vi "Dashboard Main.vi"() -> ()   [LabVIEW 2023]
uses:
  <vilib>/event_ctls.llb/eventvkey.ctl
  <vilib>/Rock Robotics/Network Tables/NT Read Numeric Array.vi
  <vilib>/Rock Robotics/WPI/Dashboard/WPI_DashboardLogging Global.vi
panel:
  in  "Camera Settings Right":T1={"Frame Rate"=30, "Compression"=30, "Size"=1, "DB Camera Config"=FALSE} {"Frame Rate" scale=1.0..30.0; "Compression" scale=100.0..-1.0; "Size" items=["640x480", "320x240", "160x120"]}
  in  "Camera Name Right":string(combo)="No Camera Selection"
  out "Camera Perf":string
  in  "Camera Settings":T1={"Frame Rate"=30, "Compression"=30, "Size"=1, "DB Camera Config"=FALSE} {"Frame Rate" scale=1.0..30.0; "Compression" scale=100.0..-1.0; "Size" items=["640x480", "320x240", "160x120"]}
  in  "TCP":refnum<k5>
  in  "Rec Mode":enum32{"Stop", "Record", "Playback"}(radio)
  out "Robot IP":string
  out "Image Message":string="Timeout in Camera Communications"
  in  "Dashboard Tab":T2(tab)
  in  "Select Auto":string(combo)="Select Autonomous ..."
  out "NT Connection":bool
  out "MotorChart R":cluster{"Numeric":dbl, "Numeric":dbl}(graph)
  out "MotorChart L":cluster{"Numeric":dbl, "Numeric":dbl}(graph)
  out "MotorSliders R":cluster{"MotorSlide1":dbl, "MotorSlide2":dbl} {"MotorSlide2" scale=-1.0..1.0 scale format="%#_2e"; "MotorSlide1" scale=-1.0..1.0 scale format="%#_2e"}
  out "MotorSliders L":cluster{"MotorSlide1":dbl, "MotorSlide2":dbl} {"MotorSlide2" scale=-1.0..1.0 scale format="%#_2e"; "MotorSlide1" scale=-1.0..1.0 scale format="%#_2e"}
  out "Encoder":dbl(knob) scale=0.0..360.0
  out "JS1 Z":dbl(slide) scale=-1.0..1.0 scale format="%#_2e"
  out "JS1 Graph":cluster{"X":dbl, "Y":dbl}[](graph)
  out "JS1 Buttons":T3
  out "JS2 Z":dbl(slide) scale=-1.0..1.0 scale format="%#_2e"
  out "JS2 Graph":cluster{"X":dbl, "Y":dbl}[](graph)
  out "JS2 Buttons":T3
  out "Mode":T4(ring)=enum."Auto Disabled"
  out "Right Camera Perf":cluster{"Bandwidth (Mbps)":dbl, "FPS":dbl}
  out "Camera Image Right":T5(plugin-control)
  in  "DB/String 9":string
  in  "DB/String 8":string
  in  "DB/String 7":string
  in  "DB/String 6":string
  in  "DB/String 5":string
  in  "DB/String 4":string
  in  "DB/String 3":string
  in  "DB/String 2":string
  in  "DB/String 1":string
  in  "DB/String 0":string
  in  "DB/Slider 0":dbl(slide) scale=0.0..5.0
  in  "DB/Slider 1":dbl(slide) scale=0.0..5.0
  in  "DB/Slider 2":dbl(slide) scale=0.0..5.0
  in  "DB/Slider 3":dbl(slide) scale=0.0..5.0
  out "DB/LED 3":bool
  out "DB/LED 2":bool
  out "DB/LED 1":bool
  out "DB/LED 0":bool
  in  "DB/Button 3":bool
  in  "DB/Button 2":bool
  in  "DB/Button 1":bool
  in  "DB/Button 0":bool caption="New Name"
  out "valorMotorEncoder":dbl
  out "encoderPsAlga":dbl(knob) scale=0.0..360.0
  in  "Test Slider":dbl(slide) scale=0.0..100.0 scale format="%#_3g"
  in  "On/Off":bool caption="Solenoid"
  in  "Test Name":u16(ring) items=["Select the test to run..."]
  in  "Test Tree":string(tree)
  in  "Motor":cluster{"Value":dbl, "Enable":bool} {"Value" scale=-1.0..1.0 scale format="%#_3g"}
  out "Progress":T6 {"Test Progress" scale=0.0..100.0}
  in  "Rev/Fwd":cluster{"Forward":bool, "Reverse":bool}
  in  "Test Ring":u16(ring) items=["Monochrome", "Color"]
  in  "CheckList":i32(listbox)
  out "Tree":string(tree)
  out "Camera Image":T5(plugin-control)
  out "Background":bool
  in  "Camera Name":string(combo)="No Camera Selection"
  # "HW"
  # "HW"
  # "Joysticks"
  # "Motores"
  # "Front"
  # "Right"
  # "Left"
  # "Back"
  # "Encoder"
  # "Valor do encoder (dado em rotações)"
  # "Valor do motor"
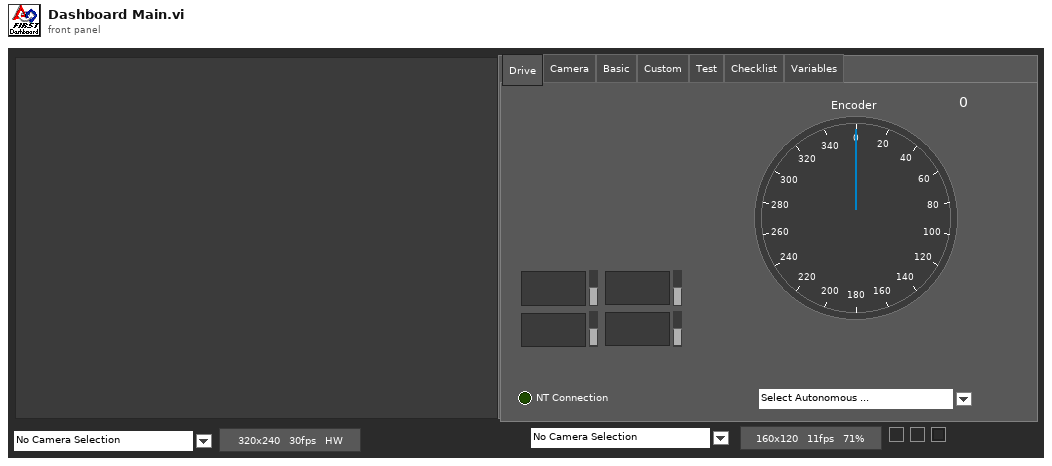
[diagram p1: front panel]
types:
  T1 = cluster{"Frame Rate":i32, "Compression":i32, "Size":u16, "DB Camera Config":bool}
  T2 = enum32{"Drive", "Camera", "Basic", "Custom", "Test", "Checklist", "Variables"}
  T3 = cluster{bool, bool, bool, bool, bool, bool, bool, bool, bool, bool, bool, bool}
  T4 = enum8{"Tele-Op Disabled", "Tele-Op Enabled", "Auto Disabled", "Auto Enabled", "Test Disabled", "Test Enabled", "Disconnected", "No Code", "E-Stop"}
  T5 = typedef "IMAQ Image.ctl" = refnum<image>
  T6 = cluster{"Test Progress":u8, "Test Progress Text":string}
  T7 = cluster{"Save Path":path, "Interval (s)":dbl, "Keep":i32}
  T8 = enum32{"Drive", "Camera", "Basic", "Custom", "Test", "Commands", "Checklist", "Variables"}
  T9 = typedef "Image Type" = u32
  T10 = cluster{"Error Strings":string, "Disable Counts":cluster{u16, u16}, "Rail Faults":cluster{u16, u16, u16}, "Robot IP":string, "DB Mode":u8, "Event Info":cluster{"Name":string, "Type":u8, "Number":u16, "Replay":u8}}
  T11 = cluster{"Storage":cluster{"Disk Free":u64, "RAM Block":u32, "RAM free":u32}, "CPU Utilization":cluster{"CPU % ISR":sgl, "CPU % Time Crit":sgl, "CPU % Timed Str":sgl, "CPU % High":sgl, "CPU % Above":sgl, "CPU % Normal":sgl, "CPU % Low":sgl}, "CAN":cluster{"% Bus Utilization":sgl, "Bus Off Cnt":u32, "TX_FIFO Full Cnt":u32, "Receive Error Cnt":u8, "Transmit Error Cnt":u8}, "HID":cluster{"HID Outputs":u32, "Rumble Low":u16, "Rumble High":u16}[]}
  T12 = cluster{"Status bits":cluster{"Test Mode":bool, "Autonomous":bool, "Enabled":bool, "Code Start":bool, "Brownout":bool, "Reserved 2":bool, "Reserved 3":bool, "E-Stop":bool}, "Code Trace":cluster{"Disabled":bool, "TeleOp":bool, "Auto":bool, "Test":bool}, "Controller Type":enum16{"unknown", "cRIO", "roboRio"}, "Code?":enum16{"unknown", "noCode", "code"}, "Battery V":dbl}
  T13 = cluster{"Control Bits":cluster{"TestMode":bool, "Autonomous":bool, "Enabled":bool, "FMS Present":bool, bool, bool, bool, "E-Stop":bool}, "Team Station ":u8, "Countdown":sgl, "Joystick Values":cluster{"Axes":dbl[], "Buttons":bool[], "POVs":i16[]}[]}
  T14 = cluster{"Axes":dbl[], "Buttons":bool[], "POVs":i16[]}[]
  T15 = cluster{"Axes":dbl[], "Buttons":bool[], "POVs":i16[]}
  T16 = cluster{"Buttons[0]":bool, "Buttons[1]":bool, "Buttons[2]":bool, "Buttons[3]":bool, "Buttons[4]":bool, "Buttons[5]":bool, "Buttons[6]":bool, "Buttons[7]":bool, "Buttons[8]":bool, "Buttons[9]":bool, "Buttons[10]":bool, "Buttons[11]":bool}
  T17 = cluster{"Camera Image":refnum<vi>, "Dashboard Tab":refnum<vi>, "Background":refnum<vi>, "Rec Mode":refnum<vi>, "Test Slider":refnum<vi>, "On/Off ":refnum<vi>, "Test Ring":refnum<vi>, "Rev/Fwd":refnum<vi>, "Test Name":refnum<vi>, "Motor":refnum<vi>, "Progress":refnum<vi>, "CheckList":refnum<vi>, "Tree":refnum<vi>, "Test Tree":refnum<vi>, "Camera Settings":refnum<vi>, "Camera Name":refnum<vi>, "Camera Perf":refnum<vi>, "Camera Settings Right":refnum<vi>, "Camera Name Right":refnum<vi>, "Camera Image Right":refnum<vi>}
  T18 = cluster{"Global Rectangle":i32[], "Contours":cluster{"Contour Type":u32, "ROI Type":u32, "Points":i32[]}[]}
  T19 = cluster{"Camera Name":string, string, "Saved DB Images Info":cluster{"Save Path":path, "Interval (s)":dbl, "Keep":i32}}
  T20 = cluster{"Camera Name Right":string, string, "Saved DB Images Info":cluster{"Save Path":path, "Interval (s)":dbl, "Keep":i32}}
  T21 = cluster{"Operation":enum16{"Update", "Clear"}, "Color Box":u32}[]
  T22 = typedef "eventvkey.ctl" = enum16{"ASCII", "Enter", "Return", "Shift", "Ctrl", "Alt", "Cmd", "Opt", "Caps", "NumLock", "Clear", "Break", "Up", "Down", "Left", "Right", "Insert", "Delete", "Home", "End", "PageUp", "PageDown", "Escape", "Help", "Pause", "ScrollLock", "F1", "F2", "F3", "F4", "F5", "F6", "F7", "F8", "F9", "F10", "F11", "F12", "F13", "F14", "F15", "F16", "F17", "F18", "F19", "F20", "F21", "F22", "F23", "F24", "Play", "VolumeUp", "VolumeDown", "Mute", "Two Byte Char"}
  T23 = cluster{"Image Size":bool, "Image Type":bool, "Pixel Value":bool, "ROI Information":bool, "Zoom Factor":bool}
  T24 = cluster{"Operation":enum16{"Update", "Clear"}, "Color Box":u32}
  T25 = cluster{"Shift":bool, "Ctrl":bool, "Alt":bool, "Cmd":bool, "Opt":bool}
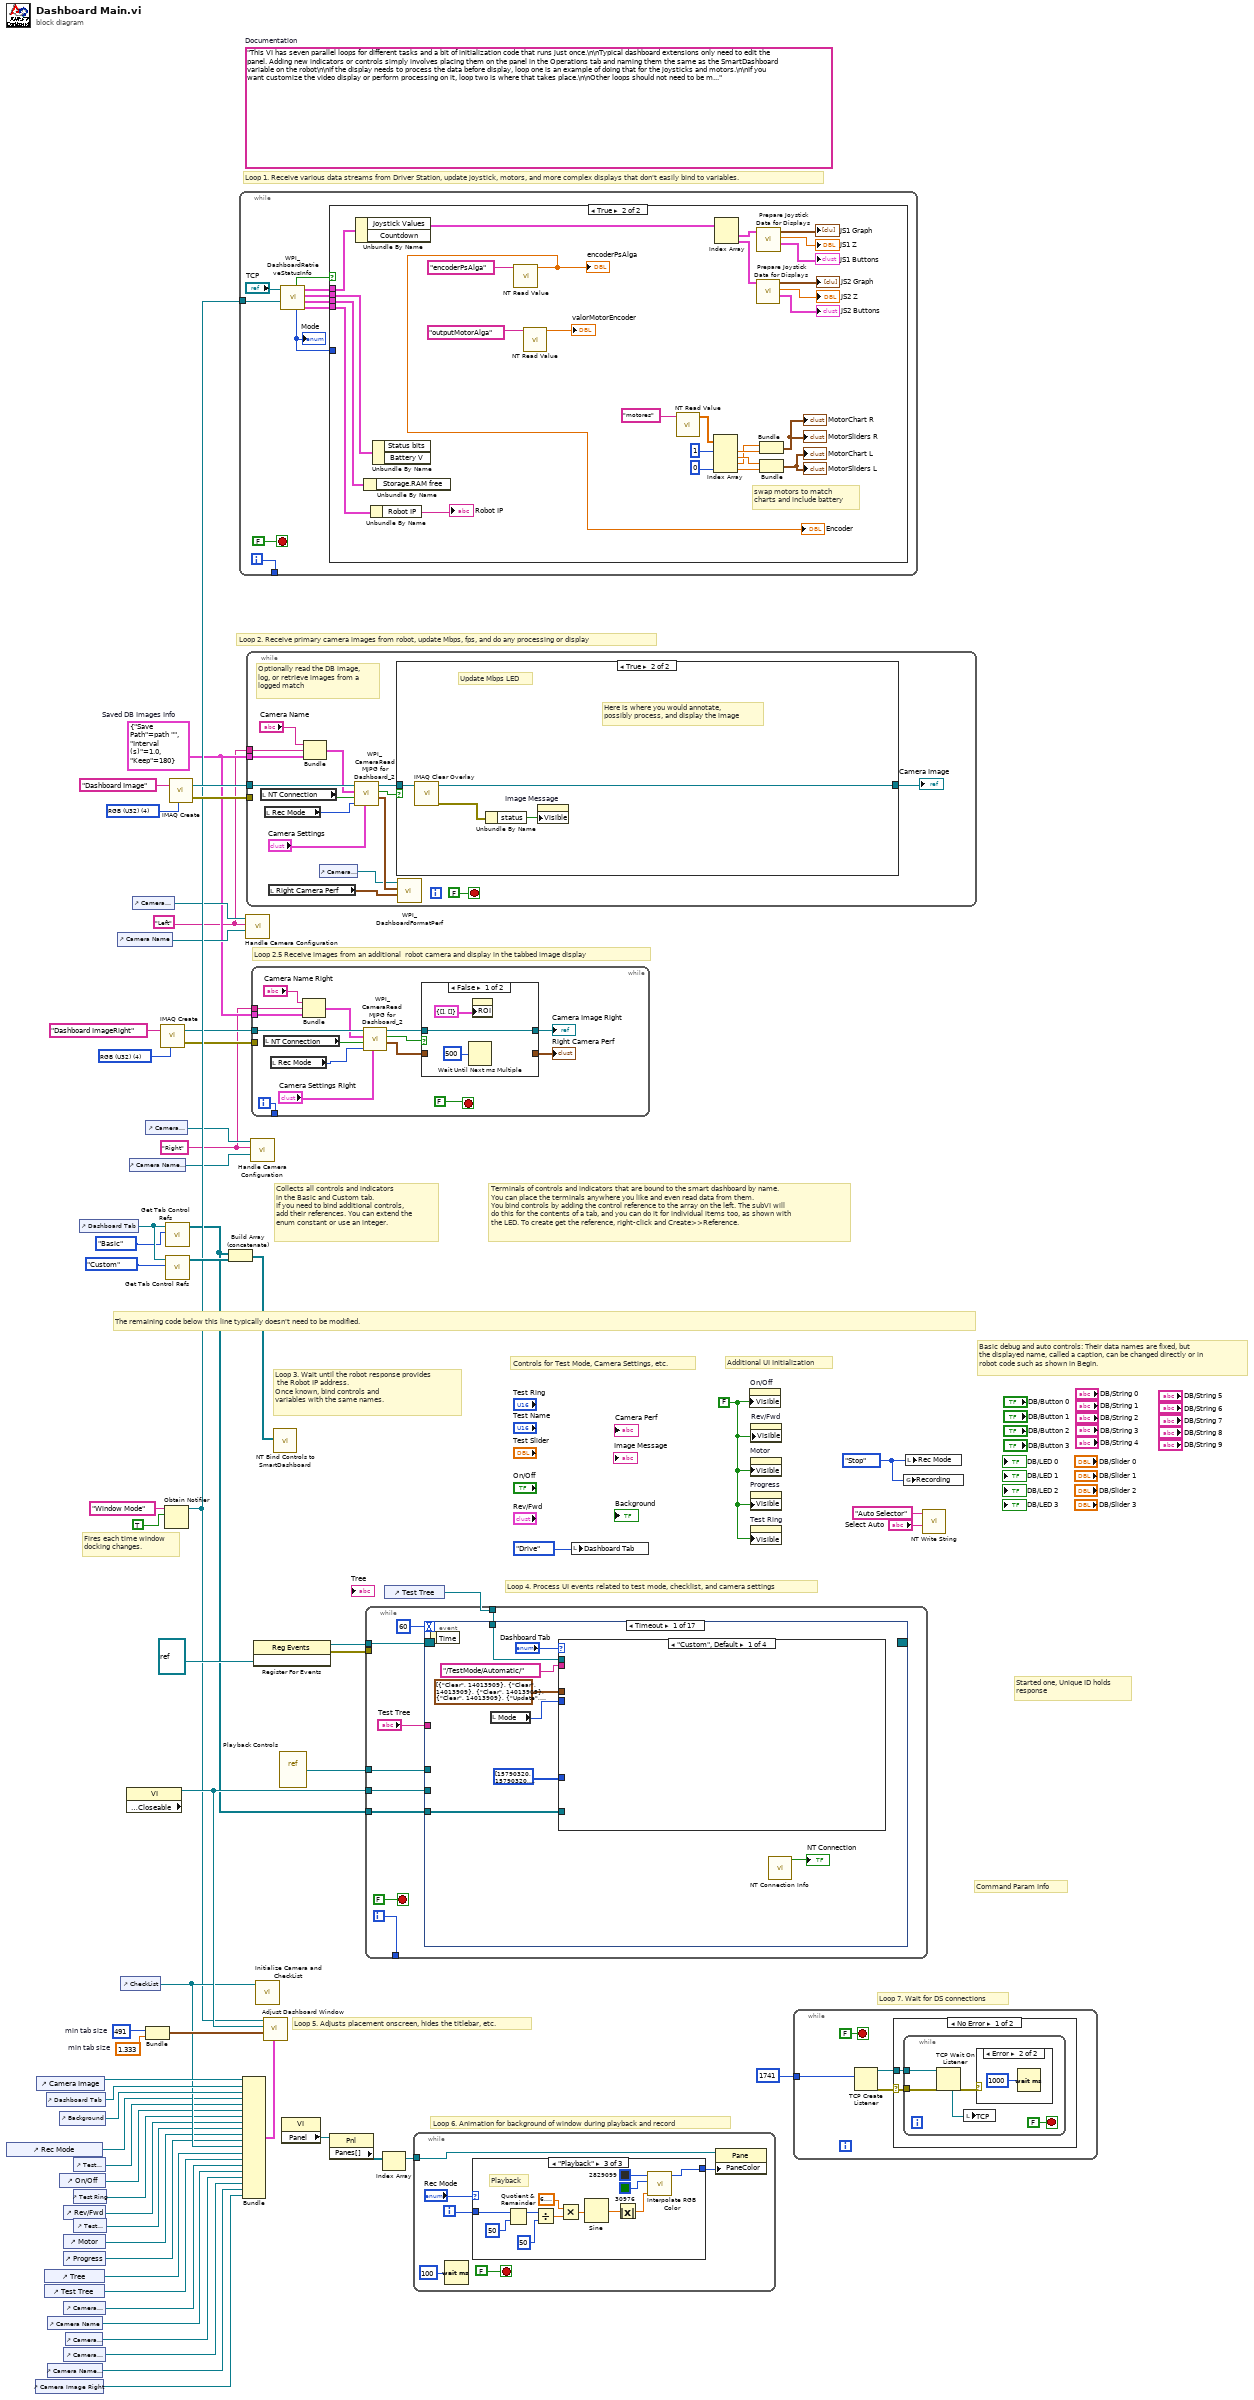
[diagram p0: block diagram]
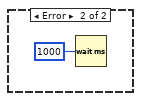
[diagram p4: hidden frame]
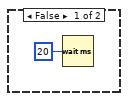
[diagram p5: hidden frame]
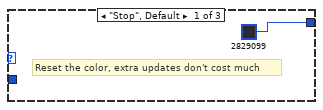
[diagram p6: hidden frame]
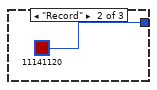
[diagram p7: hidden frame]
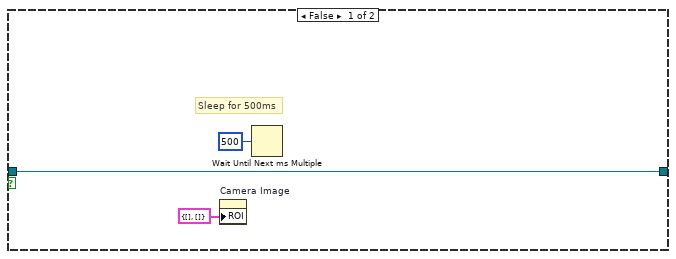
[diagram p8: hidden frame]
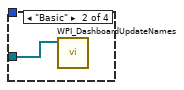
[diagram p9: hidden frame]
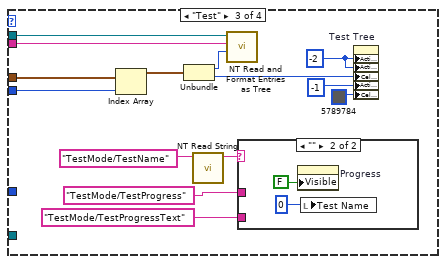
[diagram p10: hidden frame]
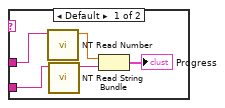
[diagram p11: hidden frame]
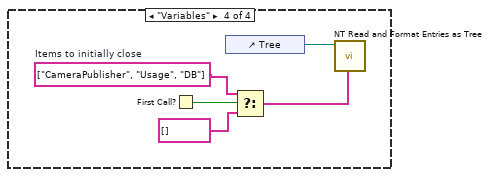
[diagram p12: hidden frame]
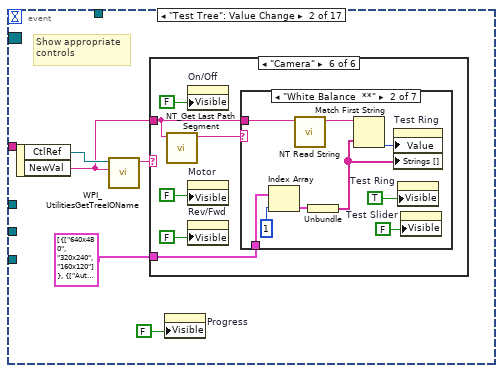
[diagram p13: hidden frame]
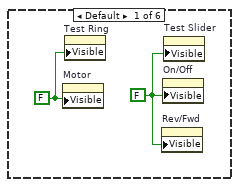
[diagram p14: hidden frame]
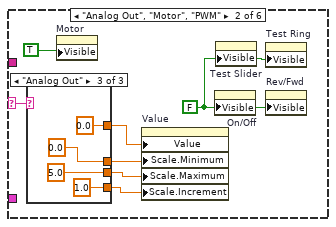
[diagram p15: hidden frame]
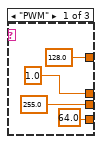
[diagram p16: hidden frame]
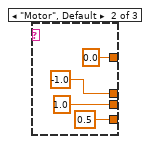
[diagram p17: hidden frame]
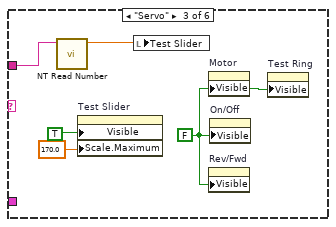
[diagram p18: hidden frame]
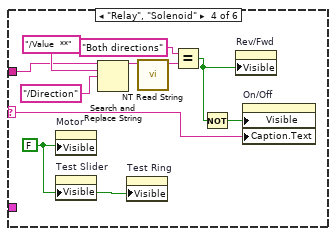
[diagram p19: hidden frame]
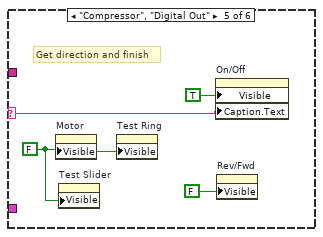
[diagram p20: hidden frame]
diagram:
  w3 = T7 {"Save Path"=path "", "Interval (s)"=1.0, "Keep"=180}  # Saved DB Images Info
  w2 = "Right"
  w1 = "Left"
  w13 = T9 4 items=["Grayscale (U8)", "Grayscale (I16)", "Grayscale (SGL)", "Complex (CSG)", "RGB (U32)", "HSL (U32)", "RGB (U64)"] ("Image Type")
  w42 = 491  # min tab size
  w41 = 1.333  # min tab size
  w49 = enum32{"Stop", "Record", "Playback"}."Stop" ("Rec Mode")
  w26 = FALSE ("Visible")
  (unwired) "This VI has seven parallel loops for different tasks and a bit of initialization code that runs just once.\n\nTypical dashboard extensions only need to edit the panel. Adding new indicators or controls simply involves placing them on the panel in the Operations tab and naming them the same as the SmartDashboard variable on the robot\n\nIf the display needs to process the data before display, loop one is an example of doing that for the joysticks and motors.\n\nIf you want customize the video display or perform processing on it, loop two is where that takes place.\n\nOther loops should not need to be modified. They are pretty standard, and document the task they perform."  # Documentation
  w63 = T9 4 items=["Grayscale (U8)", "Grayscale (I16)", "Grayscale (SGL)", "Complex (CSG)", "RGB (U32)", "HSL (U32)", "RGB (U64)"] ("Image Type")
  # "Loop 2.5 Receive images from an additional  robot camera and display in the tabbed image display"
  # "Command Param Info"
  # "Started one, Unique ID holds\nresponse"
  # "Loop 7. Wait for DS connections"
  # "Basic debug and auto controls: Their data names are fixed, but\nthe displayed name, called a caption, can be changed directly or in\nrobot code such as shown in Begin."
  # "Controls for Test Mode, Camera Settings, etc."
  # "Additional UI Initialization"
  # "Loop 6. Animation for background of window during playback and record"
  # "Fires each time window\ndocking changes."
  # "Collects all controls and indicators\nin the Basic and Custom tab.\nIf you need to bind additional controls,\nadd their references. You can extend the\nenum constant or use an integer."
  # "The remaining code below this line typically doesn't need to be modified."
  # "Loop 4. Process UI events related to test mode, checklist, and camera settings"
  # "Terminals of controls and indicators that are bound to the smart dashboard by name.\nYou can place the terminals anywhere you like and even read data from them.\nYou bind controls by adding the control reference to the array on the left. The subVI will\ndo this for the contents of a tab, and you can do it for individual items too, as shown with\nthe LED. To create get the reference, right-click and Create>>Reference."
  # "Loop 3. Wait until the robot response provides\n the Robot IP address.\nOnce known, bind controls and\nvariables with the same names."
  # "Loop 5. Adjusts placement onscreen, hides the titlebar, etc."
  # "Loop 1. Receive various data streams from Driver Station, update joystick, motors, and more complex displays that don't easily bind to variables."
  # "Loop 2. Receive primary camera images from robot, update Mbps, fps, and do any processing or display"
  n1 = control-ref of="Rec Mode"() -> (w32:refnum<vi>)
  n2 = control-ref of="Camera Image Right"() -> (w6:refnum<vi>)
  n3 = control-ref of="Camera Image"() -> (w44:refnum<vi>)
  n4 = control-ref of="Tree"() -> (w36:refnum<vi>)
  n5 = control-ref of="Test Tree"() -> (w35:refnum<vi>)
  n6 = control-ref of="Dashboard Tab"() -> (w43:refnum<vi>)
  n7 = control-ref of="Camera Name"() -> (w19:refnum<vi>)
  n8 = control-ref of="Camera Name Right"() -> (w7:refnum<vi>)
  n9 = control-ref of="Background"() -> (w39:refnum<vi>)
  n10 = control-ref of="On/Off"() -> (w30:refnum<vi>)
  n11 = control-ref of="Progress"() -> (w27:refnum<vi>)
  n12 = control-ref of="Camera Settings"() -> (w20:refnum<vi>)
  n13 = control-ref of="Camera Settings Right"() -> (w8:refnum<vi>)
  n14 = control-ref of="Rev/Fwd"() -> (w28:refnum<vi>)
  n15 = control-ref of="Motor"() -> (w33:refnum<vi>)
  n16 = control-ref of="Camera Perf"() -> (w18:refnum<vi>)
  n17 = control-ref of="Test Slider"() -> (w31:refnum<vi>)
  n18 = control-ref of="Test Ring"() -> (w29:refnum<vi>)
  n19 = control-ref of="Test Name"() -> (w34:refnum<vi>)
  n20 = control-ref of="Dashboard Tab"() -> (w47:refnum<vi>)
  n21 = control-ref of="Camera Name"() -> (w21:refnum<vi>)
  n22 = control-ref of="CheckList"() -> (w37:refnum<vi>)
  n23 = property class="VI" props=["Front Panel.Closeable"]() -> (reference out=w48:refnum<vi>)  [unwired: 2 in, 2 out]
  n24 = control-ref of="Camera Name Right"() -> (w9:refnum<vi>)
  n25 = control-ref of="Camera Settings"() -> (w22:refnum<vi>)
  n26 = control-ref of="Camera Settings Right"() -> (w10:refnum<vi>)
  n27 = Bundle("min tab size"=w42, "min tab size"=w41) -> (w40:cluster{"min tab size":i32, "min tab size":dbl})  [unwired: 1 in]
  n28 = call "IMAQ Create"("Image Name"="Dashboard ImageRight", "Image Type"=w13) -> ("New Image"=w12:T5, "error out"=w11:errorcluster)  [unwired: 2 in, 1 out]
  n29 = Obtain Notifier(name (unnamed)="Window Mode", notification data type=TRUE) -> (notifier out=w25:refnum<notifier>)  [unwired: 2 in, 2 out]
  n30 = call <vilib>:"Get Tab Control Refs.vi"("Page Index"=T8."Basic" ("Dashboard Tab"), "TabControl in"=w47) -> ("ControlsOnPage"=w17:refnum<vi>[])  [unwired: 9 in]
  n31 = call <vilib>:"Get Tab Control Refs.vi"("Page Index"=T8."Custom" ("Dashboard Tab"), "TabControl in"=w47) -> ("ControlsOnPage"=w46:refnum<vi>[])  [unwired: 9 in]
  n32 = call "IMAQ Create"("Image Name"="Dashboard Image", "Image Type"=w63) -> ("New Image"=w61:T5, "error out"=w60:errorcluster)  [unwired: 2 in, 1 out]
  n33 = Build Array (concatenate)(w17, w46) -> (w45:refnum<vi>[])
  n34 = while {
    tunnel: [w72] -> _
    tunnel: w25 -> [w64]
    i -> [w72]
    stop <- FALSE stop-if-true
    n35 = call <vilib>:"WPI_DashboardRetrieveStatusInfo.vi"("Window Mode Notifier"=w64, "TCP Cnx"="TCP") -> ("Power and Errors"=w67:T10, "Robot Metrics"=w70:T11, "Status Info"=w71:T12, "Control Info"=w68:T13, "Robot Mode"=w66:T4, "Process?"=w69:bool)  [unwired: 4 in]
    "Mode" <- w66
    n36 = case shown="True" w69 {
      tunnel: w71 -> [_ w102]
      tunnel: w70 -> [_ w101]
      tunnel: w68 -> [_ w100]
      tunnel: w67 -> [_ w99]
      tunnel: w66 -> [_ _]
      frame False {
        n37 = Wait (ms)(milliseconds to wait=u32 20) -> ()  [unwired: 1 out]
      }
      frame True {
        # "swap motors to match\ncharts and include battery"
        n38 = Unbundle By Name(w100) -> ("Joystick Values"=w90:T14)  [unwired: 1 out]
        n39 = Unbundle By Name(w101) -> ()  [unwired: 1 out]
        n40 = Unbundle By Name(w99) -> ("Robot IP"=→"Robot IP":string)
        n41 = Unbundle By Name(w102) -> ()  [unwired: 2 out]
        n42 = call-poly <vilib>:"NT Read Value.vi"("name"="encoderPsAlga") -> ("value"=→"Encoder" →"encoderPsAlga":dbl)  [unwired: 8 in, 2 out]
        n43 = call-poly <vilib>:"NT Read Value.vi"("name"="outputMotorAlga") -> ("value"=→"valorMotorEncoder":dbl)  [unwired: 8 in, 2 out]
        n44 = call-poly <vilib>:"NT Read Value.vi"("name"="motores" ("Name")) -> ("value"=w80:dbl[])  [unwired: 8 in, 2 out]
        n45 = Index Array(array=w80, index #1=1, index #4=0) -> (element #1=w94:dbl, element #2=w95:dbl, element #3=w93:dbl, element #4=w98:dbl)  [unwired: 2 in]
        n46 = Index Array(array=w90) -> (element #1=w89:T15, element #2=w85:T15)  [unwired: 2 in]
        n47 = call "Prepare Joystick Data for Displays.vi"("Joystick Values"=w85) -> ("Buttons"=→"JS2 Buttons":T16, "Z Axis"=→"JS2 Z":dbl, "Cartesian Data"=→"JS2 Graph":cluster{"X axis":dbl, "X axis":dbl}[])  [unwired: 8 in]
        n48 = call "Prepare Joystick Data for Displays.vi"("Joystick Values"=w89) -> ("Buttons"=→"JS1 Buttons":T16, "Z Axis"=→"JS1 Z":dbl, "Cartesian Data"=→"JS1 Graph":cluster{"X axis":dbl, "X axis":dbl}[])  [unwired: 8 in]
        n49 = Bundle("Numeric"=w93, "Numeric"=w94) -> (→"MotorChart R" →"MotorSliders R":cluster{"Numeric":dbl, "Numeric":dbl})  [unwired: 1 in]
        n50 = Bundle("Numeric"=w95, "Numeric"=w98) -> (→"MotorChart L" →"MotorSliders L":cluster{"Numeric":dbl, "Numeric":dbl})  [unwired: 1 in]
      }
    }
  }
  n51 = Bundle("Camera Image"=w44, "Dashboard Tab"=w43, "Background"=w39, "Rec Mode"=w32, "Test Slider"=w31, "On/Off"=w30, "Test Ring"=w29, "Rev/Fwd"=w28, "Test Name"=w34, "Motor"=w33, "Progress"=w27, "CheckList"=w37, "Tree"=w36, "Test Tree"=w35, "Camera Settings"=w20, "Camera Name"=w19, "Camera Perf"=w18, "Camera Settings Right"=w8, "Camera Name Right"=w7, "Camera Image Right"=w6) -> (w38:T17)  [unwired: 1 in]
  n52 = call "Handle Camera Configuration.vi"("CameraNameRef"=w21, "Display Name"=w1, "ClusterRef"=w22) -> ()  [unwired: 9 in]
  n53 = while {
    tunnel: w61 -> [w116]
    tunnel: w60 -> [_]
    tunnel: w3 -> [w109]
    tunnel: w1 -> [w106]
    stop <- FALSE stop-if-true
    # "Optionally read the DB image,\nlog, or retrieve images from a\nlogged match"
    n54 = local read "NT Connection"() -> (w110:bool)
    n55 = local read "Rec Mode"() -> (w113:enum32{"Stop", "Record", "Playback"})
    n56 = local read "Right Camera Perf"() -> (w104:cluster{"Bandwidth (Mbps)":dbl, "FPS":dbl})
    n57 = Bundle("Camera Name"="Camera Name", w106, "Saved DB Images Info"=w109) -> (w108:T19)  [unwired: 1 in]
    n58 = control-ref of="Camera Perf"() -> (w103:refnum<vi>)
    n59 = call <vilib>:"WPI_CameraRead MJPG for Dashboard_2.vi"("Camera Settings"="Camera Settings", "Rec Mode"=w113, "NT Connection"=w110, "Capture Info"=w108, "Image in"=w116) -> ("perf info"=w105:cluster{"Bandwidth (Mbps)":dbl, "fps":dbl}, "Active"=w114:bool, "Image\\ out"=w115:T5)  [unwired: 4 in]
    n60 = case shown="True" w114 {
      tunnel: w115 -> [w119 w122]
      tunnel: [w119 w121] -> w111
      frame False {
        # "Sleep for 500ms"
        n61 = property on="Camera Image" class="ImageControl"("ROI"=T18 {"Global Rectangle"=[], "Contours"=[]}) -> ()  [unwired: 2 in, 2 out]
        n62 = Wait Until Next ms Multiple(millisecond multiple=u32 500) -> ()  [unwired: 1 out]
      }
      frame True {
        # "Here is where you would annotate,\npossibly process, and display the image"
        # "Update Mbps LED"
        n63 = call "IMAQ Clear Overlay"("Image"=w122) -> ("error out"=w123:errorcluster, "Image Out"=w121:T5)  [unwired: 2 in, 7 out]
        n64 = Unbundle By Name(w123) -> ("status"=w124:bool)
        n65 = property on="Image Message" class="Str"("Visible"=w124) -> ()  [unwired: 2 in, 2 out]
      }
    }
    "Camera Image" <- w111
    n66 = call <vilib>:"WPI_DashboardFormatPerf.vi"("Right Camera Perf"=w104, "Performance"=w105, "String in"=w103) -> ()  [unwired: 9 in]
  }
  n67 = call "Handle Camera Configuration.vi"("CameraNameRef"=w9, "Display Name"=w2, "ClusterRef"=w10) -> ()  [unwired: 9 in]
  n68 = while {
    tunnel: w12 -> [w139]
    tunnel: w11 -> [_]
    tunnel: [w134] -> _
    tunnel: w3 -> [w130]
    tunnel: w2 -> [w127]
    i -> [w134]
    stop <- FALSE stop-if-true
    n69 = local read "NT Connection"() -> (w131:bool)
    n70 = local read "Rec Mode"() -> (w138:enum32{"Stop", "Record", "Playback"})
    n71 = Bundle("Camera Name Right"="Camera Name Right", w127, "Saved DB Images Info"=w130) -> (w129:T20)  [unwired: 1 in]
    n72 = call <vilib>:"WPI_CameraRead MJPG for Dashboard_2.vi"("Camera Settings"="Camera Settings Right", "Rec Mode"=w138, "NT Connection"=w131, "Capture Info"=w129, "Image in"=w139) -> ("perf info"=w125:cluster{"Bandwidth (Mbps)":dbl, "fps":dbl}, "Active"=w133:bool, "Image\\ out"=w136:T5)  [unwired: 4 in]
    n73 = case shown="False" w133 {
      tunnel: w136 -> [w141 w144]
      tunnel: [w141 w144] -> w132
      tunnel: [_ w143] -> w126
      tunnel: w125 -> [_ w143]
      frame False {
        n74 = Wait Until Next ms Multiple(millisecond multiple=u32 500) -> ()  [unwired: 1 out]
        n75 = property on="Camera Image Right" class="ImageControl"("ROI"=T18 {"Global Rectangle"=[], "Contours"=[]}) -> ()  [unwired: 2 in, 2 out]
      }
      frame True {
      }
    }
    "Camera Image Right" <- w132
    "Right Camera Perf" <- w126
  }
  n76 = register-events(refnum<vi> refnum) -> (reference out=w52:refnum<event-registration>, error out=w51:errorcluster)  [unwired: 2 in]
  n77 = call "Initialize Camera and CheckList.vi"("ListBox in"=w37) -> ()  [unwired: 11 in]
  n78 = call "Adjust Dashboard Window.vi"("Sizing Refnums"=w38, "Size Constraints"=w40, "VI"=w48, "WIn Mode"=w25) -> ()  [unwired: 8 in]
  n79 = call <vilib>:"NT Bind Controls to SmartDashboard.vi"("Bound Control Refs"=w45) -> ()  [unwired: 11 in]
  n80 = vi-ref "Playback Controls.vi"() -> (w53:refnum<vi>)
  n81 = property class="VI"() -> ("Panel"=w55:refnum<vi>)  [unwired: 2 in, 2 out]
  n82 = property class="Pnl"(reference=w55) -> ("Panes[]"=w56:refnum<vi>[])  [unwired: 1 in, 2 out]
  n83 = Index Array(array=w56) -> (element=w54:refnum<vi>)  [unwired: 1 in]
  n84 = control-ref of="Test Tree"() -> (w57:refnum<vi>)
  n85 = while {
    tunnel: [w150] -> _
    tunnel: w57 -> [w149]
    tunnel: w53 -> [w148]
    tunnel: w52 -> [w147]
    tunnel: w51 -> [_]
    tunnel: w48 -> [w146]
    tunnel: w17 -> [w145]
    i -> [w150]
    stop <- FALSE stop-if-true
    n86 = event shown="[0] Timeout" {
      selector: w147 -> [_ _ _ _ _ _ _ _ _ _ _ _ _ _ _ _ _]
      dyn-events: [_ _ _ _ _ _ _ _ _ _ _ _ _ w355 _ _ _] -> _
      timeout: u32 60 ("milliseconds to wait") -> [_ _ _ _ _ _ _ _ _ _ _ _ _ _ _ _ _]
      tunnel: w149 -> [w160 _ _ _ _ _ _ _ _ _ _ _ _ _ _ _ _]
      tunnel: "Test Tree" -> [_ _ _ _ _ _ _ _ w328 w335 w336 w339 w346 _ _ _ _]
      tunnel: w148 -> [_ _ _ _ _ _ _ _ _ _ _ _ _ w357 _ w372 _]
      tunnel: w146 -> [_ _ _ _ _ _ _ _ _ _ _ _ _ w353 _ _ _]
      tunnel: w145 -> [w155 _ _ _ _ _ _ _ _ _ _ _ _ _ _ _ _]
      event Timeout {
        n87 = event-data() -> ()  [unwired: 1 in, 1 out]
        n88 = local read "Mode"() -> (w158:T4)
        n89 = case shown="\"Custom\", Default" "Dashboard Tab" {
          tunnel: w160 -> [_ _ w176 _]
          tunnel: "/TestMode/Automatic/" ("Name Pattern") -> [_ _ w175 _]
          tunnel: T21 [{"Operation"=enum."Clear", "Color Box"=14013909}, {"Operation"=enum."Clear", "Color Box"=14013909}, {"Operation"=enum."Clear", "Color Box"=14013909}, {"Operation"=enum."Clear", "Color Box"=14013909}, {"Operation"=enum."Update", "Color Box"=14013909}, {"Operation"=enum."Update", "Color Box"=16777215}, {"Operation"=enum."Clear", "Color Box"=14013909}, {"Operation"=enum."Clear", "Color Box"=14013909}, {"Operation"=enum."Clear", "Color Box"=14013909}] -> [_ _ w168 _]
          tunnel: w158 -> [_ _ w167 _]
          tunnel: u32[] [15790320, 15790320, 15790320, 15790320, 16777215, 16777215, 15790320, 15790320, 15790320] -> [_ _ _ _]
          tunnel: w155 -> [_ w162 _ _]
          frame "Custom", Default {
          }
          frame "Basic" {
            n90 = call <vilib>:"WPI_DashboardUpdateNames.vi"("Controls on Tab"=w162) -> ()  [unwired: 11 in]
          }
          frame "Test" {
            w174 = -2 ("Active Item:Row Number")
            n91 = Index Array(array=w168, index=w167) -> (element=w169:T24)
            n92 = Unbundle(w169) -> ("Operation"=w170:enum16{"Update", "Clear"}, "Color Box"=w171:u32)
            n93 = call <vilib>:"NT Read String.vi"("name"="TestMode/TestName" ("Name")) -> ("value"=w165:string)  [unwired: 8 in, 2 out]
            n94 = call <vilib>:"NT Read and Format Entries as Tree.vi"("Operation"=w170, "Name Pattern"=w175, "Tree Refnum"=w176) -> ()  [unwired: 7 in, 2 out]
            n95 = case shown="\"\"" w165 {
              tunnel: "TestMode/TestProgress" ("Name") -> [w178 _]
              tunnel: "TestMode/TestProgressText" ("Name") -> [w177 _]
              frame Default {
                n96 = call <vilib>:"NT Read Number.vi"("name"=w178) -> ("value"=w179:dbl)  [unwired: 8 in, 2 out]
                n97 = call <vilib>:"NT Read String.vi"("name"=w177) -> ("value"=w180:string)  [unwired: 8 in, 2 out]
                n98 = Bundle("value"=w179, "value"=w180) -> (→"Progress":cluster{"value":dbl, "value":string})  [unwired: 1 in]
              }
              frame "" {
                n99 = property on="Progress" class="Clust (strict)"("Visible"=FALSE) -> ()  [unwired: 2 in, 2 out]
                n100 = local write "Test Name"(u16 0) -> ()
              }
            }
            n101 = property on="Test Tree" class="Tree (strict)"("Active Item Row Number"=w174, "ActiveColNum"=w174, "CellBG"=w171, "Active Item Row Number"=-1 ("Active Item:Row Number"), "CellBG"=u32 5789784 ("Color Box")) -> ()  [unwired: 2 in, 2 out]
          }
          frame "Variables" {
            w186 = string[] ["CameraPublisher", "Usage", "DB"]  # Items to initially close
            n102 = First Call?() -> (First Call?: T/F=w187:bool)
            n103 = control-ref of="Tree"() -> (w188:refnum<vi>)
            n104 = Select(t=w186, s=w187, f=string[] []) -> (s? t:f=w184:string[])
            n105 = call <vilib>:"NT Read and Format Entries as Tree.vi"("Tags to  Close"=w184, "Tree Refnum"=w188) -> ()  [unwired: 8 in, 2 out]
          }
        }
        n106 = call <vilib>:"NT Connection Info.vi"() -> ("Connected"=→"NT Connection":bool)  [unwired: 11 in]
      }
      event "Test Tree": Value Change {
        # "Show appropriate\ncontrols"
        n107 = event-data() -> ("CtlRef"=w192:refnum<vi>, "NewVal"=w190:string)  [unwired: 1 in]
        n108 = call <vilib>:"WPI_UtilitiesGetTreeIOName.vi"("NewVal"=w190, "TreeControl in"=w192) -> ("I/O Name"=w193:string)  [unwired: 9 in]
        n109 = case shown="\"Camera\"" w193 {
          selector: w193 -> [_ w200 _ w222 w231 _]
          tunnel: w190 -> [_ _ w219 w221 _ w238]
          tunnel: cluster{string[]}[] [{["640x480", "320x240", "160x120"]}, {["Auto", "Fixed indoor", "Fixed outdoor 1", "Fixed outdoor 2", "Fixed fluorescent 1", "Fixed fluorescent 2", "Hold current"]}, {["Auto", "Flicker-free 50 Hz", "Flicker-free 60 Hz", "Hold current"]}, {["None", "Prioritize frame rate", "Prioritize image quality"]}, {["Monochrome", "Color"]}] -> [_ _ _ _ _ w237]
          frame Default {
            w195 = FALSE ("Visible")
            w194 = FALSE ("Visible")
            n110 = property on="Motor" class="Clust (strict)"("Visible"=w194) -> ()  [unwired: 2 in, 2 out]
            n111 = property on="Test Ring" class="Ring (strict)"("Visible"=w194) -> ()  [unwired: 2 in, 2 out]
            n112 = property on="Rev/Fwd" class="Clust (strict)"("Visible"=w195) -> ()  [unwired: 2 in, 2 out]
            n113 = property on="On/Off" class="Bool (strict)"("Visible"=w195) -> ()  [unwired: 2 in, 2 out]
            n114 = property on="Test Slider" class="Slide (strict)"("Visible"=w195) -> ()  [unwired: 2 in, 2 out]
          }
          frame "Analog Out", "Motor", "PWM" {
            w201 = FALSE ("Visible")
            n115 = case shown="\"Analog Out\"" w200 {
              tunnel: [1.0 ("Value") -1.0 ("Value") 0.0 ("Value")] -> w199
              tunnel: [255.0 ("Value") 1.0 ("Value") 5.0 ("Value")] -> w198
              tunnel: [128.0 ("Value") 0.0 ("Value") 0.0 ("Value")] -> w197
              tunnel: [64.0 ("Value") 0.5 ("Value") 1.0 ("Value")] -> w196
              frame "PWM" {
              }
              frame "Motor", Default {
              }
              frame "Analog Out" {
              }
            }
            n116 = property on="Motor" class="Clust (strict)"("Visible"=TRUE) -> ()  [unwired: 2 in, 2 out]
            n117 = property on="Value" class="Slide (strict)"("Value"=w197, "Scale.Minimum"=w199, "Scale.Maximum"=w198, "Scale.Increment"=w196) -> ()  [unwired: 2 in, 2 out]
            n118 = property on="On/Off" class="Bool (strict)"("Visible"=w201) -> ()  [unwired: 2 in, 2 out]
            n119 = property on="Test Slider" class="Slide (strict)"("Visible"=w201) -> ()  [unwired: 2 in, 2 out]
            n120 = property on="Test Ring" class="Ring (strict)"("Visible"=w201) -> ()  [unwired: 2 in, 2 out]
            n121 = property on="Rev/Fwd" class="Clust (strict)"("Visible"=w201) -> ()  [unwired: 2 in, 2 out]
          }
          frame "Servo" {
            w217 = FALSE ("Visible")
            n122 = call <vilib>:"NT Read Number.vi"("name"=w219) -> ("value"=w218:dbl)  [unwired: 8 in, 2 out]
            n123 = property on="Test Slider" class="Slide (strict)"("Visible"=TRUE, "Scale.Maximum"=170.0 ("Scale.Range:Maximum")) -> ()  [unwired: 2 in, 2 out]
            n124 = local write "Test Slider"(w218) -> ()
            n125 = property on="Motor" class="Clust (strict)"("Visible"=w217) -> ()  [unwired: 2 in, 2 out]
            n126 = property on="Rev/Fwd" class="Clust (strict)"("Visible"=w217) -> ()  [unwired: 2 in, 2 out]
            n127 = property on="On/Off" class="Bool (strict)"("Visible"=w217) -> ()  [unwired: 2 in, 2 out]
            n128 = property on="Test Ring" class="Ring (strict)"("Visible"=w217) -> ()  [unwired: 2 in, 2 out]
          }
          frame "Relay", "Solenoid" {
            w220 = FALSE ("Visible")
            n129 = property on="Motor" class="Clust (strict)"("Visible"=w220) -> ()  [unwired: 2 in, 2 out]
            n130 = property on="Test Slider" class="Slide (strict)"("Visible"=w220) -> ()  [unwired: 2 in, 2 out]
            n131 = Search and Replace String(input string=w221, search string="/Value  **", replace string="/Direction") -> (result string=w227:string)  [unwired: 5 in, 3 out]
            n132 = property on="Test Ring" class="Ring (strict)"("Visible"=w220) -> ()  [unwired: 2 in, 2 out]
            n133 = call <vilib>:"NT Read String.vi"("name"=w227) -> ("value"=w225:string)  [unwired: 8 in, 2 out]
            n134 = Equal?(x="Both directions", y=w225) -> (x = y?=w223:bool)
            n135 = Not(x=w223) -> (.not. x?=w224:bool)
            n136 = property on="Rev/Fwd" class="Clust (strict)"("Visible"=w223) -> ()  [unwired: 2 in, 2 out]
            n137 = property on="On/Off" class="Bool (strict)"("Visible"=w224, "Caption.Text"=w222) -> ()  [unwired: 2 in, 2 out]
          }
          frame "Compressor", "Digital Out" {
            w230 = FALSE ("Visible")
            # "Get direction and finish"
            n138 = property on="Motor" class="Clust (strict)"("Visible"=w230) -> ()  [unwired: 2 in, 2 out]
            n139 = property on="Test Slider" class="Slide (strict)"("Visible"=w230) -> ()  [unwired: 2 in, 2 out]
            n140 = property on="Test Ring" class="Ring (strict)"("Visible"=w230) -> ()  [unwired: 2 in, 2 out]
            n141 = property on="On/Off" class="Bool (strict)"("Visible"=TRUE, "Caption.Text"=w231) -> ()  [unwired: 2 in, 2 out]
            n142 = property on="Rev/Fwd" class="Clust (strict)"("Visible"=FALSE) -> ()  [unwired: 2 in, 2 out]
          }
          frame "Camera" {
            n143 = call <vilib>:"NT_Get Last Path Segment.vi"("String in"=w238) -> ("String out"=w239:string)  [unwired: 10 in]
            n144 = property on="On/Off" class="Bool (strict)"("Visible"=FALSE) -> ()  [unwired: 2 in, 2 out]
            n145 = property on="Motor" class="Clust (strict)"("Visible"=FALSE) -> ()  [unwired: 2 in, 2 out]
            n146 = property on="Rev/Fwd" class="Clust (strict)"("Visible"=FALSE) -> ()  [unwired: 2 in, 2 out]
            n147 = case shown="\"White Balance  **\"" w239 {
              tunnel: w238 -> [w245 w254 w263 w272 w281 _ w287]
              tunnel: w237 -> [w243 w251 w260 w269 w278 _ _]
              frame "Size  **" {
                n148 = Index Array(array=w243) -> (element=w242:cluster{string[]})  [unwired: 1 in]
                n149 = call <vilib>:"NT Read String.vi"("name"=w245) -> ("value"=w244:string)  [unwired: 8 in, 2 out]
                n150 = Unbundle(w242) -> (w240:string[])
                n151 = Match First String(2:w240, 3:w244) -> (0:w241:i32)  [unwired: 1 out]
                n152 = property on="Test Ring" class="Ring (strict)"("Value"=w241, "Strings []"=w240) -> ()  [unwired: 2 in, 2 out]
                n153 = property on="Test Ring" class="Ring (strict)"("Visible"=TRUE) -> ()  [unwired: 2 in, 2 out]
                n154 = property on="Test Slider" class="Slide (strict)"("Visible"=FALSE) -> ()  [unwired: 2 in, 2 out]
              }
              frame "White Balance  **" {
                n155 = Index Array(array=w251, index=1) -> (element=w252:cluster{string[]})
                n156 = call <vilib>:"NT Read String.vi"("name"=w254) -> ("value"=w253:string)  [unwired: 8 in, 2 out]
                n157 = Unbundle(w252) -> (w249:string[])
                n158 = Match First String(2:w249, 3:w253) -> (0:w248:i32)  [unwired: 1 out]
                n159 = property on="Test Ring" class="Ring (strict)"("Value"=w248, "Strings []"=w249) -> ()  [unwired: 2 in, 2 out]
                n160 = property on="Test Ring" class="Ring (strict)"("Visible"=TRUE) -> ()  [unwired: 2 in, 2 out]
                n161 = property on="Test Slider" class="Slide (strict)"("Visible"=FALSE) -> ()  [unwired: 2 in, 2 out]
              }
              frame "Exposure  **" {
                n162 = Index Array(array=w260, index=2) -> (element=w261:cluster{string[]})
                n163 = call <vilib>:"NT Read String.vi"("name"=w263) -> ("value"=w262:string)  [unwired: 8 in, 2 out]
                n164 = Unbundle(w261) -> (w257:string[])
                n165 = Match First String(2:w257, 3:w262) -> (0:w258:i32)  [unwired: 1 out]
                n166 = property on="Test Ring" class="Ring (strict)"("Value"=w258, "Strings []"=w257) -> ()  [unwired: 2 in, 2 out]
                n167 = property on="Test Ring" class="Ring (strict)"("Visible"=TRUE) -> ()  [unwired: 2 in, 2 out]
                n168 = property on="Test Slider" class="Slide (strict)"("Visible"=FALSE) -> ()  [unwired: 2 in, 2 out]
              }
              frame "Exposure Priority  **" {
                n169 = Index Array(array=w269, index=3) -> (element=w270:cluster{string[]})
                n170 = call <vilib>:"NT Read String.vi"("name"=w272) -> ("value"=w271:string)  [unwired: 8 in, 2 out]
                n171 = Unbundle(w270) -> (w266:string[])
                n172 = Match First String(2:w266, 3:w271) -> (0:w267:i32)  [unwired: 1 out]
                n173 = property on="Test Ring" class="Ring (strict)"("Value"=w267, "Strings []"=w266) -> ()  [unwired: 2 in, 2 out]
                n174 = property on="Test Ring" class="Ring (strict)"("Visible"=TRUE) -> ()  [unwired: 2 in, 2 out]
                n175 = property on="Test Slider" class="Slide (strict)"("Visible"=FALSE) -> ()  [unwired: 2 in, 2 out]
              }
              frame "Color Enable  **" {
                n176 = Index Array(array=w278, index=4) -> (element=w279:cluster{string[]})
                n177 = call <vilib>:"NT Read String.vi"("name"=w281) -> ("value"=w280:string)  [unwired: 8 in, 2 out]
                n178 = Unbundle(w279) -> (w275:string[])
                n179 = Match First String(2:w275, 3:w280) -> (0:w276:i32)  [unwired: 1 out]
                n180 = property on="Test Ring" class="Ring (strict)"("Value"=w276, "Strings []"=w275) -> ()  [unwired: 2 in, 2 out]
                n181 = property on="Test Ring" class="Ring (strict)"("Visible"=TRUE) -> ()  [unwired: 2 in, 2 out]
                n182 = property on="Test Slider" class="Slide (strict)"("Visible"=FALSE) -> ()  [unwired: 2 in, 2 out]
              }
              frame Default {
                n183 = property on="Test Ring" class="Ring (strict)"("Visible"=FALSE) -> ()  [unwired: 2 in, 2 out]
                n184 = property on="Test Slider" class="Slide (strict)"("Visible"=FALSE) -> ()  [unwired: 2 in, 2 out]
              }
              frame "Brightness  **", "Color Level  **", "Compression  **", "FPS  **", "Sharpness  **" {
                n185 = call <vilib>:"NT Read Number.vi"("name"=w287) -> ("value"=w286:dbl)  [unwired: 8 in, 2 out]
                n186 = local write "Test Slider"(w286) -> ()
                n187 = property on="Test Ring" class="Ring (strict)"("Visible"=FALSE) -> ()  [unwired: 2 in, 2 out]
                n188 = property on="Test Slider" class="Slide (strict)"("Visible"=TRUE, "Scale.Maximum"=100.0 ("Scale.Range:Maximum")) -> ()  [unwired: 2 in, 2 out]
              }
            }
          }
        }
        n189 = property on="Progress" class="Clust (strict)"("Visible"=FALSE) -> ()  [unwired: 2 in, 2 out]
      }
      event "Test Name": Mouse Enter {
        # "Populate the ring with the list of tests"
        n190 = event-data() -> ()  [unwired: 1 in, 1 out]
        n191 = call <vilib>:"NT Read String Array.vi"("name"="TestMode/TestList" ("Name")) -> ("value"=w294:string[])  [unwired: 8 in, 2 out]
        n192 = Build Array (concatenate)("Select the test to run...", w294) -> (w293:string[])
        n193 = property on="Test Name" class="Ring (strict)"("Strings []"=w293) -> ()  [unwired: 2 in, 2 out]
      }
      event "Test Name": Value Change {
        w295 = FALSE ("Visible")
        # "Tell the robot the test name to run"
        n194 = event-data() -> ("NewVal"=w299:u16)  [unwired: 1 in]
        n195 = property on="Test Name" class="Ring (strict)"() -> ("Strings []"=w300:string[])  [unwired: 2 in, 2 out]
        n196 = local write "Progress"(T6 {"Test Progress"=0, "Test Progress Text"=""} ("Progress")) -> ()
        n197 = Index Array(array=w300, index=w299) -> (element=w298:string)
        n198 = call <vilib>:"NT Write String.vi"("value"=w298, "name"="TestMode/TestName" ("Name")) -> ()  [unwired: 9 in, 1 out]
        n199 = property on="Progress" class="Clust (strict)"("Visible"=TRUE) -> ()  [unwired: 2 in, 2 out]
        n200 = property on="Motor" class="Clust (strict)"("Visible"=w295) -> ()  [unwired: 2 in, 2 out]
        n201 = property on="Test Slider" class="Slide (strict)"("Visible"=w295) -> ()  [unwired: 2 in, 2 out]
        n202 = property on="On/Off" class="Bool (strict)"("Visible"=w295) -> ()  [unwired: 2 in, 2 out]
        n203 = property on="Rev/Fwd" class="Clust (strict)"("Visible"=w295) -> ()  [unwired: 2 in, 2 out]
        n204 = property on="Test Ring" class="Ring (strict)"("Visible"=w295) -> ()  [unwired: 2 in, 2 out]
      }
      event "Select Auto": Mouse Enter {
        # "Populate the combo box with the list of autonomous options"
        n205 = event-data() -> ()  [unwired: 1 in, 1 out]
        n206 = call <vilib>:"NT Read String Array.vi"("name"="Auto List" ("Name")) -> ("value"=w302:string[])  [unwired: 8 in, 2 out]
        n207 = property on="Select Auto" class="CmbBox"("Strings[]"=w302) -> ()  [unwired: 2 in, 2 out]
      }
      event "Select Auto": Value Change {
        # "User modified the Auto Selection. Write to NT variable so robot knows."
        n208 = event-data() -> ("NewVal"=w304:string)  [unwired: 1 in]
        n209 = call <vilib>:"NT Write String.vi"("value"=w304, "name"="Auto Selector" ("Name")) -> ()  [unwired: 9 in, 1 out]
      }
      event "CheckList": Double Click {
        # "Shift clears all"
        # "Update symbols on the listbox"
        n210 = event-data() -> ("PlatMods.Shift"=w306:bool, "Row"=w308:i32)  [unwired: 1 in]
        n211 = case shown="True" w306 {
          tunnel: w308 -> [w312 _]
          tunnel: 1 -> [w311 _]
          frame False {
            n212 = property on="CheckList" class="LstBox (strict)"() -> ("Item Symbols"=w310:i32[])  [unwired: 2 in, 2 out]
            n213 = Replace Array Subset(array=w310, new element=w311, index=w312) -> (w309:i32[])
            n214 = property on="CheckList" class="LstBox (strict)"("Item Symbols"=w309) -> ()  [unwired: 2 in, 2 out]
          }
          frame True {
            w313 = 0 ("Top Row")
            n215 = property on="CheckList" class="LstBox (strict)"() -> ("Number of Rows"=w315:u32)  [unwired: 2 in, 2 out]
            n216 = Initialize Array(0, w315) -> (w314:i32[])
            n217 = property on="CheckList" class="LstBox (strict)"("Top Row"=w313, "Value"=w313, "Item Symbols"=w314) -> ()  [unwired: 2 in, 2 out]
          }
        }
      }
      event "CheckList": Key Down {
        # "Update symbols on the listbox\nLeft and right keys check and uncheck"
        n218 = event-data() -> ("VKey"=w318:T22)  [unwired: 1 in]
        n219 = case shown="\"Left\", \"Right\"" w318 {
          selector: w318 -> [w323 _]
          tunnel: eventvkey."Left" ("VKey") -> [w321 _]
          frame "Left", "Right" {
            n220 = Equal?(x=w321, y=w323) -> (x = y?=w322:bool)
            n221 = Select(t=0, s=w322, f=1) -> (s? t:f=w324:i32)
            n222 = property on="CheckList" class="LstBox (strict)"() -> ("Item Symbols"=w327:i32[])  [unwired: 2 in, 2 out]
            n223 = Replace Array Subset(array=w327, new element=w324, index="CheckList") -> (w326:i32[])
            n224 = property on="CheckList" class="LstBox (strict)"("Item Symbols"=w326) -> ()  [unwired: 2 in, 2 out]
          }
          frame Default {
          }
        }
      }
      event "Motor.Enable": Value Change {
        # "When the test mode otor enable helper is set, update that\ntree row item's value"
        n225 = event-data() -> ("NewVal"=w332:bool)  [unwired: 1 in]
        n226 = Unbundle("Motor") -> ("Value"=w331:dbl)  [unwired: 1 out]
        n227 = Select(t=w331, s=w332, f=0.0) -> (s? t:f=w329:dbl)
        n228 = call <vilib>:"NT Write Number.vi"("value"=w329, "name"=w328) -> ()  [unwired: 9 in, 1 out]
      }
      event "Test Slider": Value Change {
        # "When the test mode slider helper is set, update that\ntree row item's value"
        n229 = event-data() -> ("NewVal"=w334:dbl)  [unwired: 1 in]
        n230 = call <vilib>:"NT Write Number.vi"("value"=w334, "name"=w335) -> ()  [unwired: 9 in, 1 out]
      }
      event "On/Off": Value Change {
        # "When the test mode on/off helper value is set, update that\ntree row item's value"
        n231 = event-data() -> ("NewVal"=w338:bool)  [unwired: 1 in]
        n232 = Boolean To (0,1)(Boolean=w338) -> (0, 1=w337:i16)
        n233 = call <vilib>:"NT Write Number.vi"("value"=w337, "name"=w336) -> ()  [unwired: 9 in, 1 out]
      }
      event "Rev/Fwd": Value Change {
        # "When the test mode helper value for relays is set, update that\ntree row item's value"
        n234 = event-data() -> ("NewVal.Forward"=w345:bool, "NewVal.Reverse"=w344:bool)  [unwired: 1 in]
        n235 = Boolean To (0,1)(Boolean=w345) -> (0, 1=w341:i16)
        n236 = Boolean To (0,1)(Boolean=w344) -> (0, 1=w343:i16)
        n237 = Negate(x=w343) -> (-x=w342:i16)
        n238 = Add(x=w341, y=w342) -> (x+y=w340:i16)
        n239 = call <vilib>:"NT Write Number.vi"("value"=w340, "name"=w339) -> ()  [unwired: 9 in, 1 out]
      }
      event "Test Ring": Value Change {
        # "When a test mode helper value is selected from the ring,\nset the tree item's variable to the string value"
        n240 = event-data() -> ("NewVal"=w348:u16)  [unwired: 1 in]
        n241 = property on="Test Ring" class="Ring (strict)"() -> ("Strings []"=w349:string[])  [unwired: 2 in, 2 out]
        n242 = Index Array(array=w349, index=w348) -> (element=w347:string)
        n243 = call <vilib>:"NT Write String.vi"("value"=w347, "name"=w346) -> ()  [unwired: 9 in, 1 out]
      }
      event "Rec Mode": Value Change {
        # "Update globals for recording mode and path to read log from.\nClear when logging and let NetworkTables set path for vision to\nuse."
        n244 = event-data() -> ("NewVal"=w358:enum32{"Stop", "Record", "Playback"})  [unwired: 1 in]
        n245 = global write "WPI_DashboardLogging Global.vi" "Logging Filename"(path "") -> ()
        n246 = global write "WPI_DashboardLogging Global.vi" "Recording"(w358) -> ()
        n247 = case shown="\"Playback\"" w358 {
          tunnel: w357 -> [_ w360 w368]
          tunnel: [_ _ w367] -> w355
          tunnel: [_ _ w366] -> _
          tunnel: w353 -> [_ _ w364]
          tunnel: cluster{i32, i32} {-250, 170} -> [_ _ w363]
          tunnel: [_ _ T23 {"Image Size"=TRUE, "Image Type"=TRUE, "Pixel Value"=TRUE, "ROI Information"=TRUE, "Zoom Factor"=FALSE} ("Image Information Shown:All Elements")] -> w350
          tunnel: [_ _ TRUE ("Zoom Factor")] -> w351
          frame Default {
          }
          frame "Stop", "Record" {
            # "Place Window too"
            n248 = invoke class="VI" method="FP.Close"(reference=w360) -> (reference out=w359:refnum<vi>)  [unwired: 2 in, 2 out]
            n249 = invoke class="VI" method="Abort VI"(reference=w359) -> ()  [unwired: 2 in, 3 out]
          }
          frame "Playback" {
            n250 = call "Open Playback Panel.vi"("Offset"=w363, "DB VI Ref"=w364, "Playback in"=w368) -> ("Playback out"=w365:refnum<vi>)  [unwired: 8 in]
            n251 = register-events(w365) -> (reference out=w367:refnum<event-registration>, error out=w366:errorcluster)  [unwired: 2 in]
          }
        }
        n252 = property on="Camera Image Right" class="ImageControl"("Image Information Shown"=w350, "Image Information Visible"=w351) -> ()  [unwired: 2 in, 2 out]
        n253 = property on="Camera Image" class="ImageControl"("Image Information Shown"=w350, "Image Information Visible"=w351) -> ()  [unwired: 2 in, 2 out]
        n254 = call <vilib>:"WPI_DashboardNT Log FieldName Cache.vi"("Operation"=enum16{"Lookup/Add", "Index", "Clear"}."Clear") -> ()  [unwired: 8 in, 3 out]
      }
      event Panel Close {
        w369 = enum32{"Stop", "Record", "Playback"}."Stop" ("Rec Mode")
        # "Playback window has been closed, abort"
        n255 = event-data() -> ()  [unwired: 1 in, 4 out]
        n256 = local write "Rec Mode"(w369) -> ()
        n257 = global write "WPI_DashboardLogging Global.vi" "Recording"(w369) -> ()
      }
      event Panel Close {
        # "Abort playback window and ourself"
        n258 = event-data() -> ()  [unwired: 1 in, 4 out]
        n259 = invoke class="VI" method="FP.Close"(reference=w372) -> (reference out=w371:refnum<vi>)  [unwired: 2 in, 2 out]
        n260 = invoke class="VI" method="Abort VI"(reference=w371) -> (error out=w370:errorcluster)  [unwired: 2 in, 2 out]
        n261 = invoke class="VI" method="Abort VI"(error in=w370) -> ()  [unwired: 2 in, 3 out]
      }
      event "Tree": Double Click {
        n262 = event-data() -> ("PlatMods"=w378:T25, "Tag"=w375:string)  [unwired: 1 in]
        n263 = Unbundle(w378) -> ("Shift"=w377:bool)  [unwired: 4 out]
        n264 = String Subset(string=w375, length (rest)=1 ("length (rest)")) -> (substring=w374:string)  [unwired: 1 in]
        n265 = Not(x=w377) -> (.not. x?=w376:bool)
        n266 = case shown="\"/\"" w374 {
          tunnel: w375 -> [_ w380]
          tunnel: w376 -> [_ w379]
          frame Default {
          }
          frame "/" {
            n267 = call <vilib>:"NT Update Persistence.vi"("Persistence"=w379, "Name"=w380) -> ()  [unwired: 9 in, 1 out]
          }
        }
      }
    }
  }
  n268 = while {
    tunnel: w54 -> [w382]
    i -> [w385]
    stop <- FALSE stop-if-true
    n269 = Wait (ms)(milliseconds to wait=u32 100) -> ()  [unwired: 1 out]
    n270 = case shown="\"Playback\"" "Rec Mode" {
      tunnel: w385 -> [_ _ w400]
      tunnel: [u32 2829099 ("Base Color") u32 11141120 ("Target Color") w389] -> w381
      frame "Stop", Default {
        # "Reset the color, extra updates don't cost much"
      }
      frame "Record" {
      }
      frame "Playback" {
        # "Playback"
        n271 = Quotient & Remainder(x=w400, y=u32 50 ("milliseconds to wait")) -> (x-y*floor(x/y)=w396:u32)  [unwired: 1 out]
        n272 = Divide(x=w396, y=u32 50 ("milliseconds to wait")) -> (x/y=w393:dbl)
        n273 = Multiply(x=6.283185307179586, y=w393) -> (x*y=w398:dbl)
        n274 = Sine(x=w398) -> (sin(x)=w397:dbl)
        n275 = Absolute Value(x=w397) -> (abs(x)=w390:dbl)
        n276 = call "Interpolate RGB Color.vi"("Proportion"=w390, "Target Color"=u32 30976, "Base Color"=u32 2829099) -> ("Result Color"=w389:u32)  [unwired: 8 in]
      }
    }
    n277 = property class="Pane"(reference=w382, "PaneColor"=w381) -> ()  [unwired: 1 in, 2 out]
  }
  n278 = local write "Dashboard Tab"(T2."Drive" ("Dashboard Tab")) -> ()
  n279 = property on="On/Off" class="Bool (strict)"("Visible"=w26) -> ()  [unwired: 2 in, 2 out]
  n280 = property on="Motor" class="Clust (strict)"("Visible"=w26) -> ()  [unwired: 2 in, 2 out]
  n281 = property on="Progress" class="Clust (strict)"("Visible"=w26) -> ()  [unwired: 2 in, 2 out]
  n282 = property on="Test Ring" class="Ring (strict)"("Visible"=w26) -> ()  [unwired: 2 in, 2 out]
  n283 = property on="Rev/Fwd" class="Clust (strict)"("Visible"=w26) -> ()  [unwired: 2 in, 2 out]
  n284 = while {
    tunnel: u16 1741 ("timeout ms (25000)") -> [w402]
    stop <- FALSE stop-if-true
    n285 = TCP Create Listener(10:w402) -> (0:w401:errorcluster, 3:w403:refnum<k5>)  [unwired: 4 in, 1 out]
    n286 = case shown="No Error" w401 {
      selector: w401 -> [w405 _]
      tunnel: w403 -> [w406 _]
      frame No Error {
        n287 = while {
          tunnel: w406 -> [w409]
          tunnel: w405 -> [w408]
          stop <- FALSE stop-if-true
          n288 = TCP Wait On Listener(8:w408, 11:w409) -> (0:w410:errorcluster, 4:w411:refnum<k5>)  [unwired: 2 in, 3 out]
          n289 = local write "TCP"(w411) -> ()
          n290 = case shown="Error" w410 {
            frame No Error {
            }
            frame Error {
              n291 = Wait (ms)(milliseconds to wait=u32 1000) -> ()  [unwired: 1 out]
            }
          }
        }
      }
      frame Error {
        n292 = Wait (ms)(milliseconds to wait=u32 1000) -> ()  [unwired: 1 out]
      }
    }
  }
  n293 = global write "WPI_DashboardLogging Global.vi" "Recording"(w49) -> ()
  n294 = local write "Rec Mode"(w49) -> ()
  n295 = call <vilib>:"NT Write String.vi"("value"="Select Auto", "name"="Auto Selector" ("Name")) -> ()  [unwired: 9 in, 1 out]
